vi "p6100_general_setpoint.vi"   [LabVIEW 2011]
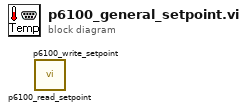
[diagram p0: block diagram]
diagram:
  n1 = call "p6100_read_setpoint.vi"() -> ()  [unwired: 5 in, 3 out]
  n2 = call "p6100_write_setpoint.vi"() -> ()  [unwired: 5 in, 3 out]
